vi "Send Single Trigger.vi"(8 "error in (no error)":errorcluster, 11 "VNA-ENA in":refnum<class "VNA-ENA.lvclass">) -> (0 "error out":errorcluster, 3 "VNA-ENA out":refnum<class "VNA-ENA.lvclass">)   [LabVIEW 2020, in "VNA-ENA.lvclass"]
doc: "Sent a single trigger for the VNA. It uses the OPC command to wait until completion.\nIt will use (sweeptime * N average * N ports) for the VISA timeout."
uses:
  VNA-ENA.lvclass
  C:/Sandbox/Git_Sandbox/WiSpry Test Framework source code (LV20)/WiSpry Test Framework/Instruments/Instrument.lvclass
  Instrument.lvclass/Instrument.ctl
  Instrument.lvclass
  <instrlib>/Agilent ENA Series/Agilent ENA Series.lvlib
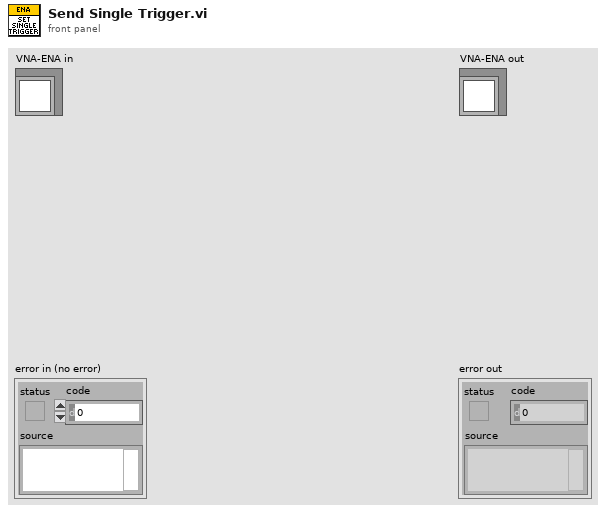
[diagram p1: front panel]
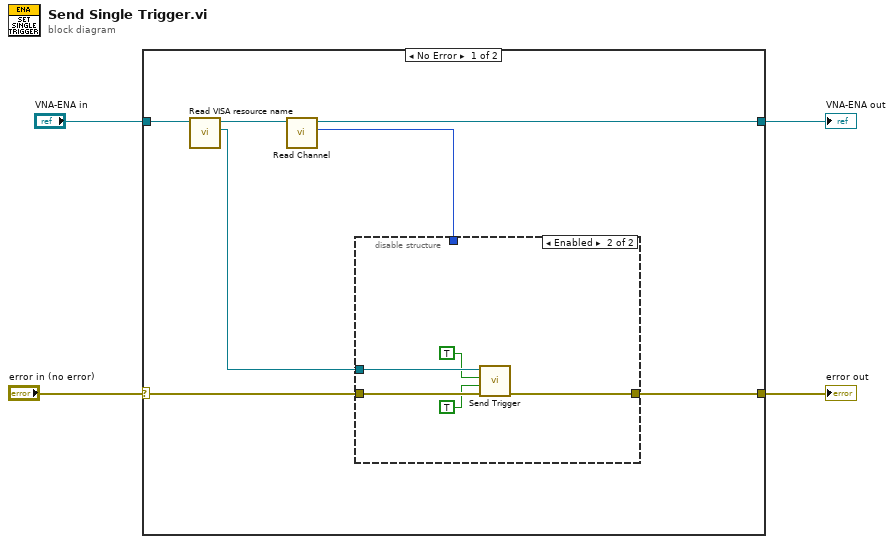
[diagram p0: block diagram]
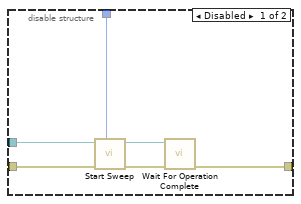
[diagram p2: hidden frame]
diagram:
  n1 = case shown="No Error" "error in (no error)" {
    selector: "error in (no error)" -> [w9 w24]
    tunnel: [w8 w24] -> w3
    tunnel: [w6 w23] -> w2
    tunnel: "VNA-ENA in" -> [w11 w23]
    frame No Error {
      n2 = call "Read VISA resource name.vi"("Instrument in"=w11) -> ("VISA resource name"=w10:refnum<visa-resource-name>, "Instrument out"=w7:refnum<class "VNA-ENA.lvclass">)  [unwired: 9 in]
      n3 = call-dynamic "Read Channel.vi"("Vector Network Analyzer in"=w7) -> ("Channel"=w5:i32, "Vector Network Analyzer out"=w6:refnum<class "VNA-ENA.lvclass">)  [unwired: 9 in]
      n4 = disable-structure shown="Enabled" {
        disable-tunnel: w10 -> [w17 w21]
        disable-tunnel: w9 -> [w16 w22]
        disable-tunnel: [w15 w18] -> w8
        disable-tunnel: w5 -> [w12 _]
        frame Disabled {
          n5 = call <instrlib>:"Start Sweep.vi"("Channel (1)"=w12, "error in (no error)"=w16, "VISA resource name"=w17) -> ("error out"=w13:errorcluster, "VISA resource name out"=w14:refnum<visa-resource-name>)  [unwired: 7 in]
          n6 = call <instrlib>:"Wait For Operation Complete.vi"("error in (no error)"=w13, "VISA resource name"=w14) -> ("error out"=w15:errorcluster)  [unwired: 8 in, 1 out]
        }
        frame Enabled {
          n7 = call <instrlib>:"Send Trigger.vi"("error in (no error)"=w22, "Wait for OPC (F: Do not Wait)"=TRUE, "Ignore Trigger Source (F: Do not Ignore)"=TRUE, "VISA resource name"=w21) -> ("error out"=w18:errorcluster)  [unwired: 6 in, 1 out]
        }
      }
    }
    frame Error {
    }
  }
  "error out" <- w3
  "VNA-ENA out" <- w2
